vi "Initialize Device Core.vi"(8 "error in (no error)":errorcluster, 9 "Reset (F)":bool, 10 "Resource Name":string, 11 "CS++Motor in":refnum<class "CS++Motor.lvclass">) -> (0 "error out":errorcluster, 3 "CS++Motor out":refnum<class "CS++Motor.lvclass">)   [LabVIEW 2015, in "CS++Motor.lvlib" / "CS++Motor.lvclass"]
doc: "Initialize device driver."
uses:
  CS++Motor.lvclass
  CSPP_Core/Classes/CS++ProcessVariables/ProcessVariable/PV.lvclass
  CS++Motor.lvclass/CS++Motor.ctl
  PV-Enum-n.ctl
  CSPP_Core/Classes/CS++ProcessVariables/ProcessVariable/PV.lvclass/PV.ctl
  CSPP_Core/Classes/CS++ProcessVariables/ProcessVariable/Write Data.vi
  CSPP_Core/Classes/CS++ProcessVariables/ProcessVariable/Write Timestamp.vi
  CSPP_Core/Classes/CS++ProcessVariables/ProcessVariable/Write Quality.vi
  CSPP_Core/Classes/CS++ProcessVariables/ProcessVariable/Write status.vi
  CSPP_Core/Actors/CS++DeviceActor/CS++DeviceActor.lvclass
  CSPP_Core/Classes/CS++ProcessVariables/PVConnection/PVConnection.lvclass
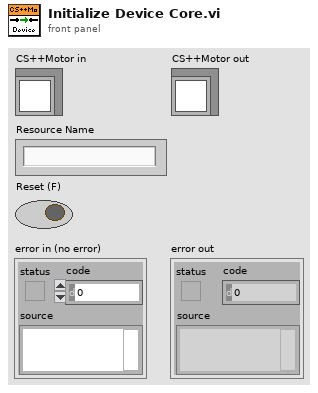
[diagram p1: front panel]
types:
  T1 = cluster{"LogicalName":string, "PhysicalName":string, "unit":string, "Scaling":dbl, "Scaling Offset":dbl, "StartVelocity":dbl, "StopVelocity":dbl, "Acceleration":dbl, "RangeMin":dbl, "RangeMax":dbl, "LogicalPos-Array":cluster{"LogicalPosition":string, "SetPosition":dbl}[]}[]
  T2 = typedef "CS++Motor.lvlib/CS++Motor.lvclass/PV-Enum-n.ctl" = enum16{"PhysicalName", "unit", "ActPosition", "SetPosition", "RawSetPosition", "StartVelocity", "StopVelocity", "Acceleration", "RangeMin", "RangeMax", "Scaling", "ScalingOffset", "RangeRefError", "LogicalPositionArray", "NoOfCommands"}
  T3 = cluster{"LogicalPosition":string, "SetPosition":dbl}[]
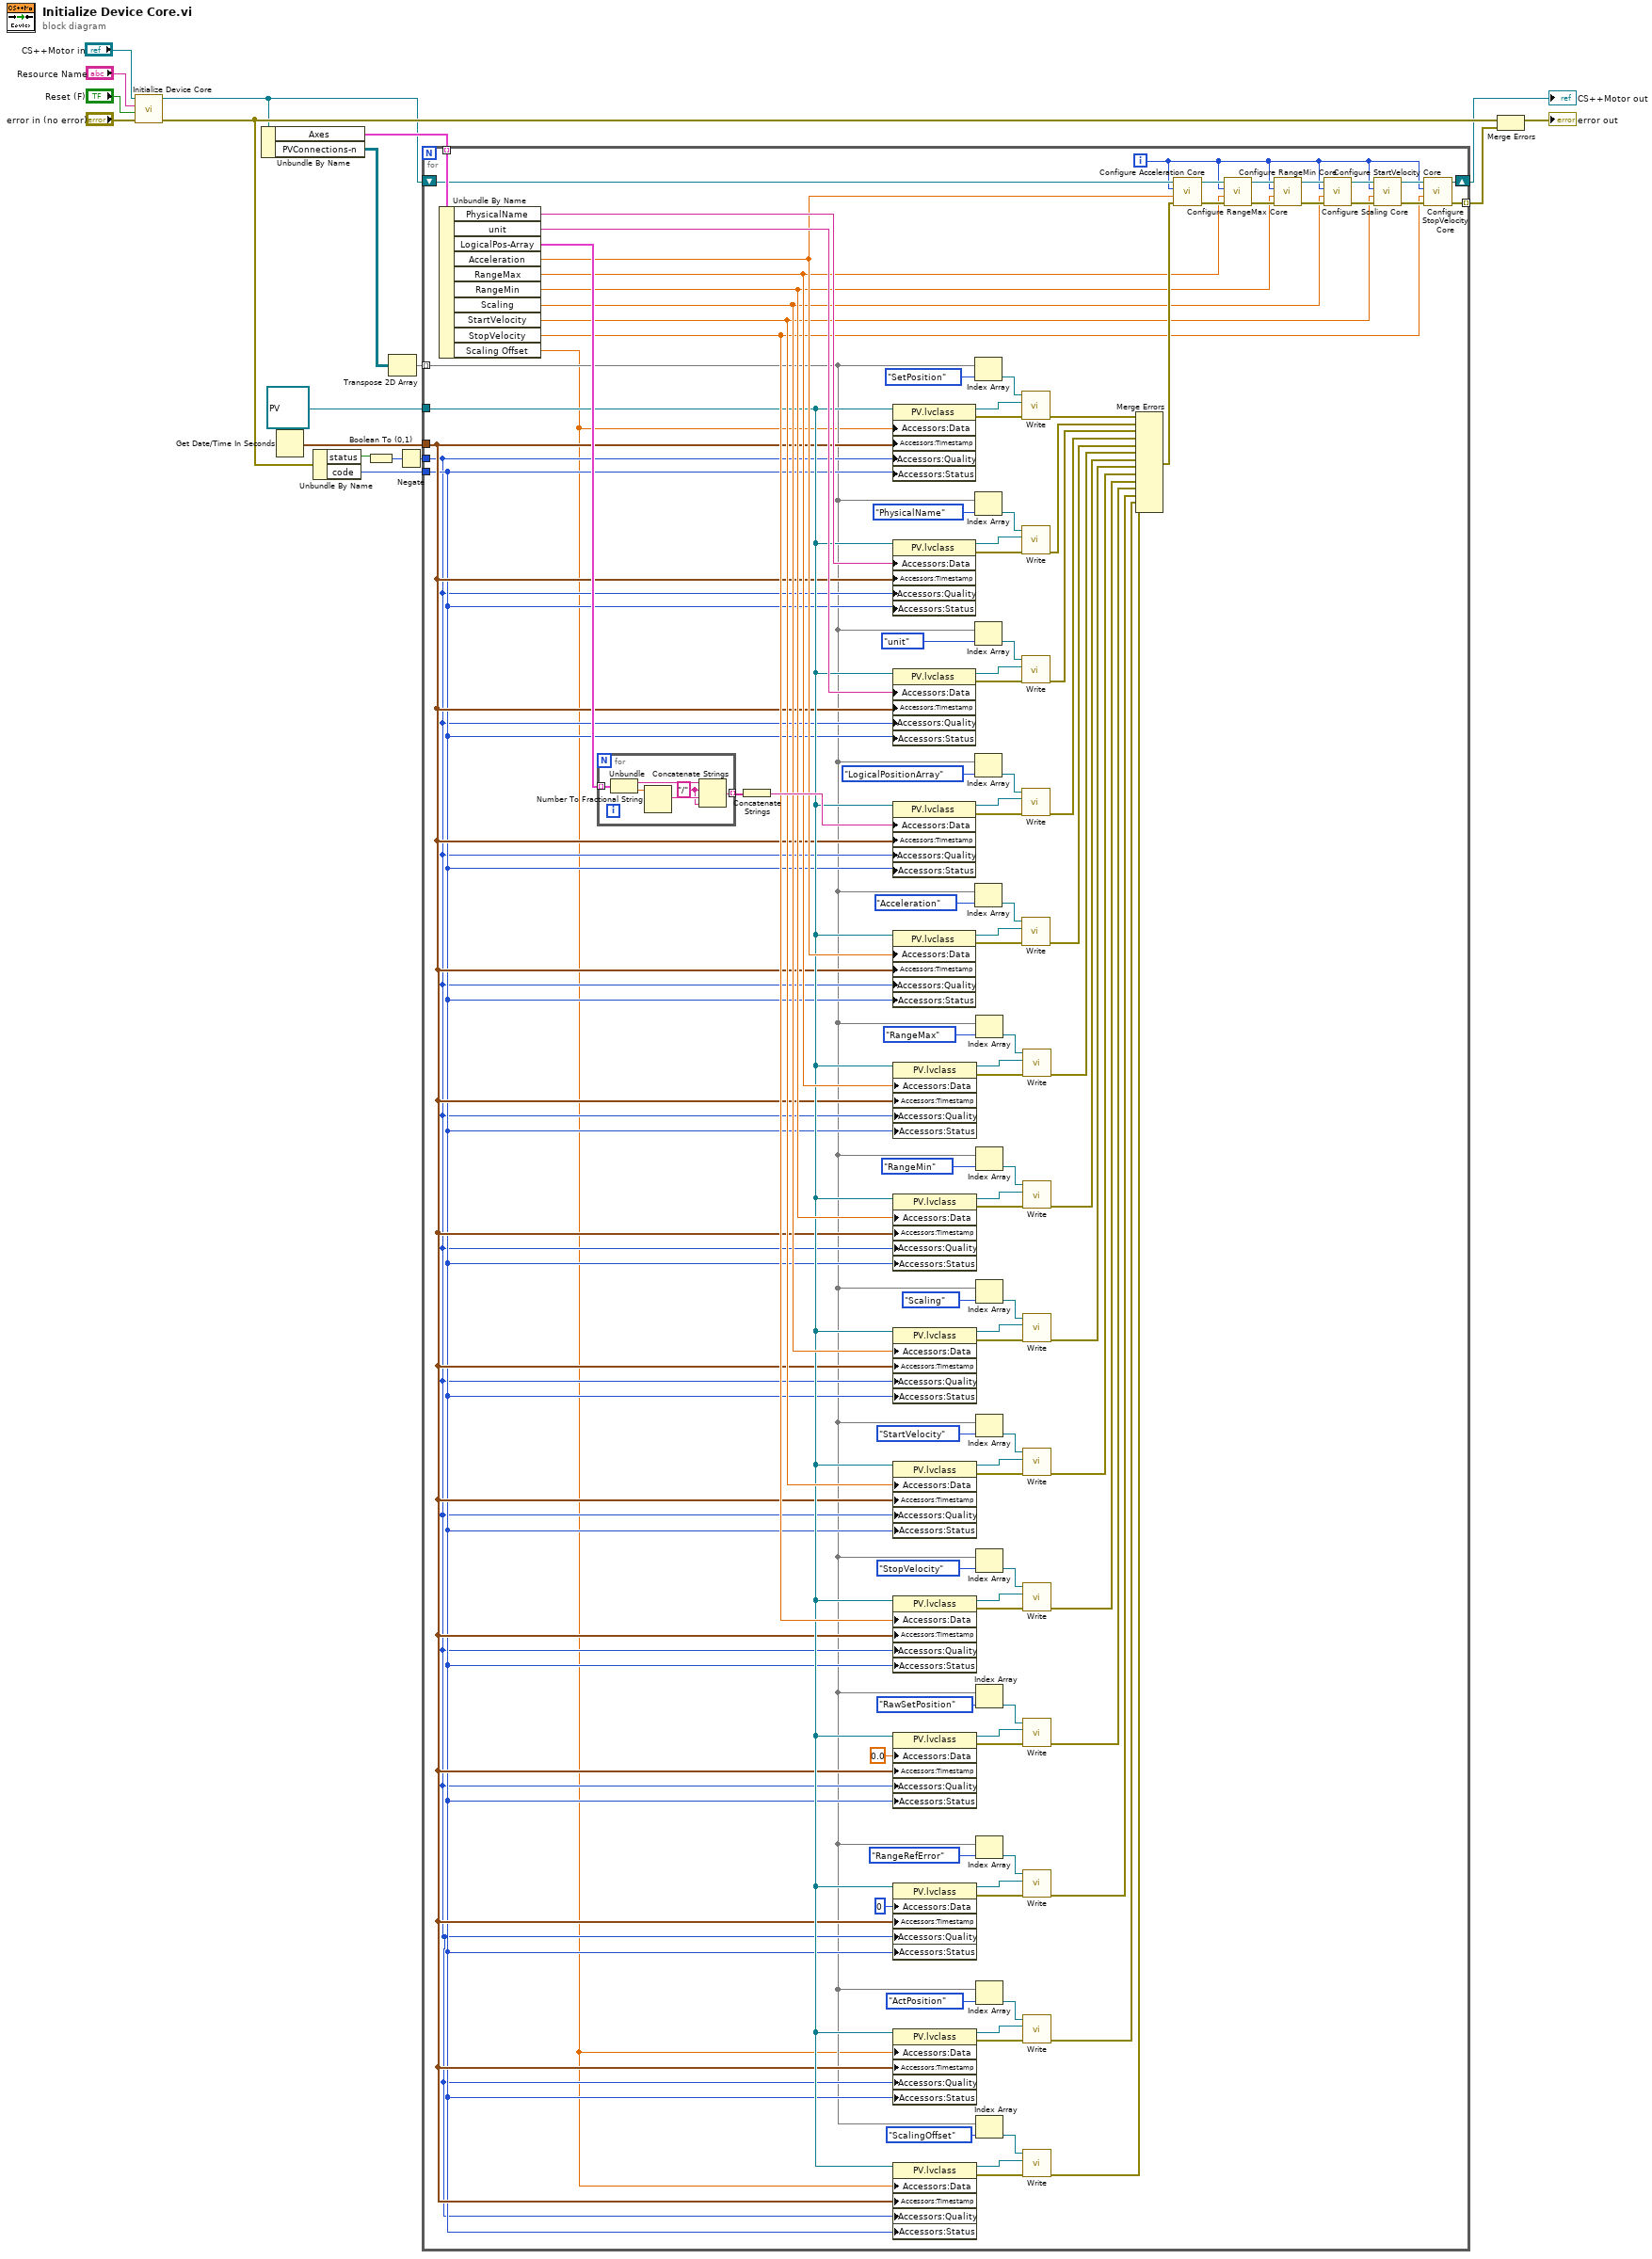
[diagram p0: block diagram]
diagram:
  n1 = call-parent "Initialize Device Core.vi"("error in (no error)"="error in (no error)", "Reset (F)"="Reset (F)", "Resource Name"="Resource Name", "CS++DeviceActor in"="CS++Motor in") -> ("error out"=w7:errorcluster, "CS++DeviceActor out"=w1:refnum<class "CS++Motor.lvclass">)  [unwired: 6 in]
  n2 = Unbundle By Name(w1) -> ("Axes"=w5:T1, "PVConnections-n"=w8:refnum<class "PVConnection.lvclass">[][])
  n3 = Get Date/Time In Seconds() -> (seconds since 1Jan1904=w14:timestamp)
  n4 = Unbundle By Name(w7) -> ("status"=w12:bool, "code"=w10:i32)
  n5 = Boolean To (0,1)(Boolean=w12) -> (0, 1=w11:i16)
  n6 = Transpose 2D Array(2D array=w8) -> (transposed array=w4:refnum<class "PVConnection.lvclass">[][])
  n7 = Negate(x=w11) -> (-x=w9:i16)
  n8 = for {
    tunnel: w14 -> [w24]
    tunnel: refnum<class "PV.lvclass"> refnum ("PV") -> [w25]
    tunnel: w10 -> [w23]
    tunnel: w9 -> [w22]
    tunnel: w4 -> [w21] mode=indexing
    tunnel: w5 -> [w117] mode=indexing
    tunnel: [w44] -> w3 mode=indexing
    shift-right: [w38] -> w2
    shift-left: w1 -> [w37]
    i -> [w36]
    n9 = Unbundle By Name(w117) -> ("PhysicalName"=w116:string, "unit"=w109:string, "LogicalPos-Array"=w63:T3, "Acceleration"=w35:dbl, "RangeMax"=w34:dbl, "RangeMin"=w33:dbl, "Scaling"=w32:dbl, "StartVelocity"=w31:dbl, "StopVelocity"=w30:dbl, "Scaling Offset"=w19:dbl)
    n10 = for {
      tunnel: w63 -> [w129] mode=indexing
      tunnel: [w124] -> w64 mode=indexing
      w125 = "/" ("string")
      n11 = Unbundle(w129) -> ("LogicalPosition"=w127:string, "SetPosition"=w128:dbl)
      n12 = Number To Fractional String(number=w128) -> (F-format string=w126:string)  [unwired: 3 in]
      n13 = Concatenate Strings(w127, w125, w126, w125) -> (w124:string)
    }
    n14 = Concatenate Strings(w64) -> (w62:string)
    n15 = property class="PV.lvclass"(reference=w25, "Accessors:Data"=w19, "Accessors:Timestamp"=w24, "Accessors:Quality"=w22, "Accessors:Status"=w23) -> (reference out=w123:refnum<class "PV.lvclass">, error out=w122:errorcluster)  [unwired: 1 in]
    n16 = property class="PV.lvclass"(reference=w25, "Accessors:Data"=w116, "Accessors:Timestamp"=w24, "Accessors:Quality"=w22, "Accessors:Status"=w23) -> (reference out=w120:refnum<class "PV.lvclass">, error out=w119:errorcluster)  [unwired: 1 in]
    n17 = property class="PV.lvclass"(reference=w25, "Accessors:Data"=w109, "Accessors:Timestamp"=w24, "Accessors:Quality"=w22, "Accessors:Status"=w23) -> (reference out=w111:refnum<class "PV.lvclass">, error out=w112:errorcluster)  [unwired: 1 in]
    n18 = property class="PV.lvclass"(reference=w25, "Accessors:Data"=w62, "Accessors:Timestamp"=w24, "Accessors:Quality"=w22, "Accessors:Status"=w23) -> (reference out=w108:refnum<class "PV.lvclass">, error out=w107:errorcluster)  [unwired: 1 in]
    n19 = property class="PV.lvclass"(reference=w25, "Accessors:Data"=w35, "Accessors:Timestamp"=w24, "Accessors:Quality"=w22, "Accessors:Status"=w23) -> (reference out=w102:refnum<class "PV.lvclass">, error out=w103:errorcluster)  [unwired: 1 in]
    n20 = property class="PV.lvclass"(reference=w25, "Accessors:Data"=w34, "Accessors:Timestamp"=w24, "Accessors:Quality"=w22, "Accessors:Status"=w23) -> (reference out=w100:refnum<class "PV.lvclass">, error out=w99:errorcluster)  [unwired: 1 in]
    n21 = property class="PV.lvclass"(reference=w25, "Accessors:Data"=w33, "Accessors:Timestamp"=w24, "Accessors:Quality"=w22, "Accessors:Status"=w23) -> (reference out=w96:refnum<class "PV.lvclass">, error out=w95:errorcluster)  [unwired: 1 in]
    n22 = property class="PV.lvclass"(reference=w25, "Accessors:Data"=w32, "Accessors:Timestamp"=w24, "Accessors:Quality"=w22, "Accessors:Status"=w23) -> (reference out=w92:refnum<class "PV.lvclass">, error out=w91:errorcluster)  [unwired: 1 in]
    n23 = property class="PV.lvclass"(reference=w25, "Accessors:Data"=w31, "Accessors:Timestamp"=w24, "Accessors:Quality"=w22, "Accessors:Status"=w23) -> (reference out=w88:refnum<class "PV.lvclass">, error out=w87:errorcluster)  [unwired: 1 in]
    n24 = property class="PV.lvclass"(reference=w25, "Accessors:Data"=w30, "Accessors:Timestamp"=w24, "Accessors:Quality"=w22, "Accessors:Status"=w23) -> (reference out=w84:refnum<class "PV.lvclass">, error out=w83:errorcluster)  [unwired: 1 in]
    n25 = property class="PV.lvclass"(reference=w25, "Accessors:Data"=0.0, "Accessors:Timestamp"=w24, "Accessors:Quality"=w22, "Accessors:Status"=w23) -> (reference out=w67:refnum<class "PV.lvclass">, error out=w68:errorcluster)  [unwired: 1 in]
    n26 = property class="PV.lvclass"(reference=w25, "Accessors:Data"=u8 0, "Accessors:Timestamp"=w24, "Accessors:Quality"=w22, "Accessors:Status"=w23) -> (reference out=w58:refnum<class "PV.lvclass">, error out=w59:errorcluster)  [unwired: 1 in]
    n27 = property class="PV.lvclass"(reference=w25, "Accessors:Data"=w19, "Accessors:Timestamp"=w24, "Accessors:Quality"=w22, "Accessors:Status"=w23) -> (reference out=w53:refnum<class "PV.lvclass">, error out=w54:errorcluster)  [unwired: 1 in]
    n28 = property class="PV.lvclass"(reference=w25, "Accessors:Data"=w19, "Accessors:Timestamp"=w24, "Accessors:Quality"=w22, "Accessors:Status"=w23) -> (reference out=w29:refnum<class "PV.lvclass">, error out=w28:errorcluster)  [unwired: 1 in]
    n29 = Index Array(array=w21, index=PV-Enum-n."SetPosition" ("PV-Enum-n")) -> (element=w121:refnum<class "PVConnection.lvclass">)
    n30 = Index Array(array=w21, index=PV-Enum-n."PhysicalName" ("PV-Enum-n")) -> (element=w118:refnum<class "PVConnection.lvclass">)
    n31 = Index Array(array=w21, index=PV-Enum-n."unit" ("PV-Enum-n")) -> (element=w113:refnum<class "PVConnection.lvclass">)
    n32 = Index Array(array=w21, index=PV-Enum-n."LogicalPositionArray" ("PV-Enum-n")) -> (element=w106:refnum<class "PVConnection.lvclass">)
    n33 = Index Array(array=w21, index=PV-Enum-n."Acceleration" ("PV-Enum-n")) -> (element=w104:refnum<class "PVConnection.lvclass">)
    n34 = Index Array(array=w21, index=PV-Enum-n."RangeMax" ("PV-Enum-n")) -> (element=w98:refnum<class "PVConnection.lvclass">)
    n35 = Index Array(array=w21, index=PV-Enum-n."RangeMin" ("PV-Enum-n")) -> (element=w94:refnum<class "PVConnection.lvclass">)
    n36 = Index Array(array=w21, index=PV-Enum-n."Scaling" ("PV-Enum-n")) -> (element=w90:refnum<class "PVConnection.lvclass">)
    n37 = Index Array(array=w21, index=PV-Enum-n."StartVelocity" ("PV-Enum-n")) -> (element=w86:refnum<class "PVConnection.lvclass">)
    n38 = Index Array(array=w21, index=PV-Enum-n."StopVelocity" ("PV-Enum-n")) -> (element=w82:refnum<class "PVConnection.lvclass">)
    n39 = Index Array(array=w21, index=PV-Enum-n."RawSetPosition" ("PV-Enum-n")) -> (element=w69:refnum<class "PVConnection.lvclass">)
    n40 = Index Array(array=w21, index=PV-Enum-n."RangeRefError" ("PV-Enum-n")) -> (element=w60:refnum<class "PVConnection.lvclass">)
    n41 = Index Array(array=w21, index=PV-Enum-n."ActPosition" ("PV-Enum-n")) -> (element=w55:refnum<class "PVConnection.lvclass">)
    n42 = Index Array(array=w21, index=PV-Enum-n."ScalingOffset" ("PV-Enum-n")) -> (element=w27:refnum<class "PVConnection.lvclass">)
    n43 = call "Write.vi"("error in (no error)"=w122, "PV"=w123, "PVConnection in"=w121) -> ("error out"=w115:errorcluster)  [unwired: 7 in, 1 out]
    n44 = call "Write.vi"("error in (no error)"=w119, "PV"=w120, "PVConnection in"=w118) -> ("error out"=w114:errorcluster)  [unwired: 7 in, 1 out]
    n45 = call "Write.vi"("error in (no error)"=w112, "PV"=w111, "PVConnection in"=w113) -> ("error out"=w110:errorcluster)  [unwired: 7 in, 1 out]
    n46 = call "Write.vi"("error in (no error)"=w107, "PV"=w108, "PVConnection in"=w106) -> ("error out"=w105:errorcluster)  [unwired: 7 in, 1 out]
    n47 = call "Write.vi"("error in (no error)"=w103, "PV"=w102, "PVConnection in"=w104) -> ("error out"=w101:errorcluster)  [unwired: 7 in, 1 out]
    n48 = call "Write.vi"("error in (no error)"=w99, "PV"=w100, "PVConnection in"=w98) -> ("error out"=w97:errorcluster)  [unwired: 7 in, 1 out]
    n49 = call "Write.vi"("error in (no error)"=w95, "PV"=w96, "PVConnection in"=w94) -> ("error out"=w93:errorcluster)  [unwired: 7 in, 1 out]
    n50 = call "Write.vi"("error in (no error)"=w91, "PV"=w92, "PVConnection in"=w90) -> ("error out"=w89:errorcluster)  [unwired: 7 in, 1 out]
    n51 = call "Write.vi"("error in (no error)"=w87, "PV"=w88, "PVConnection in"=w86) -> ("error out"=w85:errorcluster)  [unwired: 7 in, 1 out]
    n52 = call "Write.vi"("error in (no error)"=w83, "PV"=w84, "PVConnection in"=w82) -> ("error out"=w81:errorcluster)  [unwired: 7 in, 1 out]
    n53 = call "Write.vi"("error in (no error)"=w68, "PV"=w67, "PVConnection in"=w69) -> ("error out"=w65:errorcluster)  [unwired: 7 in, 1 out]
    n54 = call "Write.vi"("error in (no error)"=w59, "PV"=w58, "PVConnection in"=w60) -> ("error out"=w57:errorcluster)  [unwired: 7 in, 1 out]
    n55 = call "Write.vi"("error in (no error)"=w54, "PV"=w53, "PVConnection in"=w55) -> ("error out"=w52:errorcluster)  [unwired: 7 in, 1 out]
    n56 = call "Write.vi"("error in (no error)"=w28, "PV"=w29, "PVConnection in"=w27) -> ("error out"=w20:errorcluster)  [unwired: 7 in, 1 out]
    n57 = Merge Errors(w115, w114, w110, w105, w101, w97, w93, w89, w85, w81, w65, w57, w52, w20) -> (w50:errorcluster)
    n58 = call-dynamic "Configure Acceleration Core.vi"("error in (no error)"=w50, "Acceleration"=w35, "AxisNumber"=w36, "CS++Motor in"=w37) -> ("error out"=w49:errorcluster, "CS++Motor out"=w43:refnum<class "CS++Motor.lvclass">)  [unwired: 6 in]
    n59 = call-dynamic "Configure RangeMax Core.vi"("error in (no error)"=w49, "RangeMax"=w34, "AxisNumber"=w36, "CS++Motor in"=w43) -> ("error out"=w48:errorcluster, "CS++Motor out"=w42:refnum<class "CS++Motor.lvclass">)  [unwired: 6 in]
    n60 = call-dynamic "Configure RangeMin Core.vi"("error in (no error)"=w48, "RangeMin"=w33, "AxisNumber"=w36, "CS++Motor in"=w42) -> ("error out"=w47:errorcluster, "CS++Motor out"=w41:refnum<class "CS++Motor.lvclass">)  [unwired: 6 in]
    n61 = call-dynamic "Configure Scaling Core.vi"("error in (no error)"=w47, "Scaling"=w32, "AxisNumber"=w36, "CS++Motor in"=w41) -> ("error out"=w46:errorcluster, "CS++Motor out"=w40:refnum<class "CS++Motor.lvclass">)  [unwired: 6 in]
    n62 = call-dynamic "Configure StartVelocity Core.vi"("error in (no error)"=w46, "StartVelocity"=w31, "AxisNumber"=w36, "CS++Motor in"=w40) -> ("error out"=w45:errorcluster, "CS++Motor out"=w39:refnum<class "CS++Motor.lvclass">)  [unwired: 6 in]
    n63 = call-dynamic "Configure StopVelocity Core.vi"("error in (no error)"=w45, "StopVelocity"=w30, "AxisNumber"=w36, "CS++Motor in"=w39) -> ("error out"=w44:errorcluster, "CS++Motor out"=w38:refnum<class "CS++Motor.lvclass">)  [unwired: 6 in]
  }
  "CS++Motor out" <- w2
  n64 = Merge Errors(w7, w3) -> (→"error out":errorcluster)
